vi "Box Function.vi"(6 "Index":i32, 9 "Freq Index":u8, 10 "Signal Type":enum16{"Sine", "Square", "Triangle"}(ring), 11 "CAN Frame [Write] In":cluster{"Identifier":u32, "Data Bytes":u8[]} {"Data Bytes" format="%x"; "Identifier" format="%x"}) -> (1 "State":T1, 2 "Freq":dbl, 3 "CAN Frame [Write]":T2 {"payload" format="%x"; "timestamp" format="%<%I:%M:%S%8u %p\n%x>T"; "identifier" format="%x"})   [LabVIEW 2015]
uses:
  <vilib>/Stratom, Inc/X-CAN for myRIO (API)/X-CAN Class/Type Definitions/CANFrame.ctl
  Control/State.ctl
  <vilib>/Stratom, Inc/X-CAN for myRIO (API)/X-CAN Class/X-CAN.lvclass
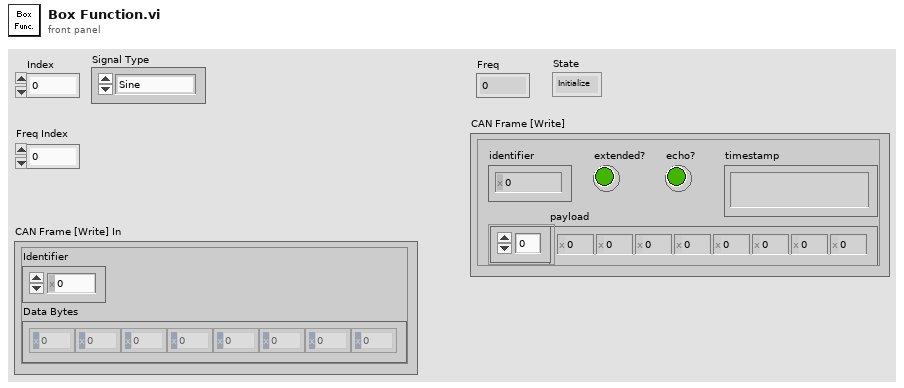
[diagram p1: front panel]
types:
  T1 = typedef "State.ctl" = enum16{"Initialize", "Idle", "Write", "Stop"}
  T2 = typedef "X-CAN.lvclass/CANFrame.ctl" = cluster{"identifier":u32, "extended?":bool, "echo?":bool, "payload":u8[], "timestamp":timestamp}
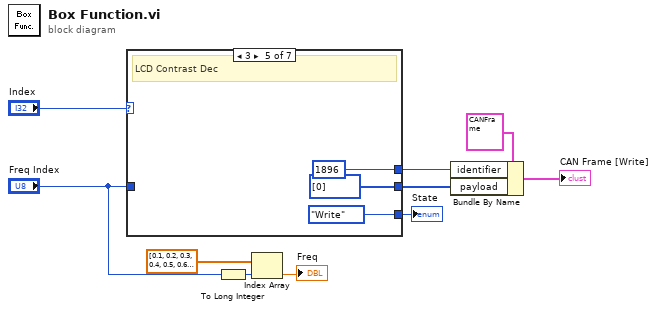
[diagram p0: block diagram]
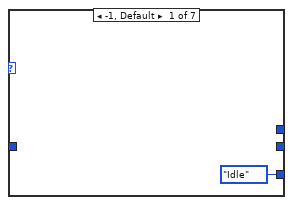
[diagram p2: hidden frame]
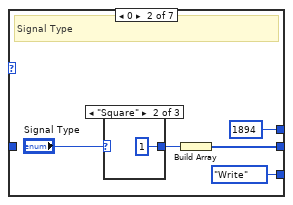
[diagram p3: hidden frame]
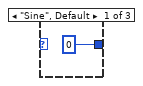
[diagram p4: hidden frame]
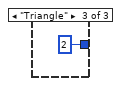
[diagram p5: hidden frame]
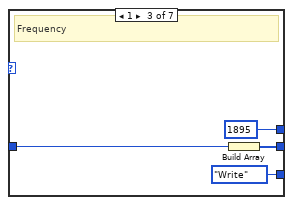
[diagram p6: hidden frame]
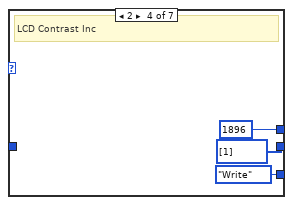
[diagram p7: hidden frame]
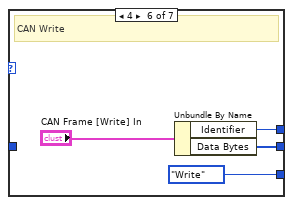
[diagram p8: hidden frame]
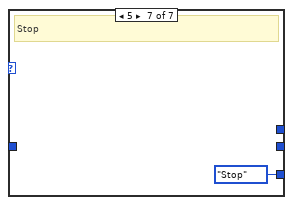
[diagram p9: hidden frame]
diagram:
  n1 = case shown="3" "Index" {
    tunnel: [_ u32 1894 u32 1895 u32 1896 u32 1896 w32 _] -> w7
    tunnel: [_ w13 w22 u8[] [1] ("Data Bytes") u8[] [0] ("Data Bytes") w31 _] -> w6
    tunnel: [State."Idle" State."Write" State."Write" State."Write" State."Write" State."Write" State."Stop"] -> w5
    tunnel: "Freq Index" -> [_ _ w20 _ _ _ _]
    frame -1, Default {
    }
    frame 0 {
      # "Signal Type"
      n2 = case shown="\"Square\"" "Signal Type" {
        tunnel: [u8 0 u8 1 u8 2] -> w14
        frame "Sine", Default {
        }
        frame "Square" {
        }
        frame "Triangle" {
        }
      }
      n3 = Build Array(w14) -> (w13:u8[])
    }
    frame 1 {
      # "Frequency"
      n4 = Build Array(w20) -> (w22:u8[])
    }
    frame 2 {
      # "LCD Contrast Inc"
    }
    frame 3 {
      # "LCD Contrast Dec"
    }
    frame 4 {
      # "CAN Write"
      n5 = Unbundle By Name("CAN Frame [Write] In") -> ("Identifier"=w32:u32, "Data Bytes"=w31:u8[])
    }
    frame 5 {
      # "Stop"
    }
  }
  "State" <- w5
  n6 = To Long Integer(number="Freq Index") -> (32bit integer=w3:i32)
  n7 = Index Array(array=dbl[] [0.1, 0.2, 0.3, 0.4, 0.5, 0.6, 0.7, 0.8, 0.9, 1.0, 2.0, 3.0, 4.0, 5.0, 6.0, 7.0, 8.0, 9.0, 10.0, 20.0, 30.0, 40.0, 50.0, 60.0, 70.0, 80.0, 90.0, 100.0, 110.0, 120.0, 130.0, 140.0, 150.0, 160.0, 170.0, 180.0, 190.0, 200.0, 210.0, 220.0, 230.0, 240.0, 250.0, 260.0, 270.0, 280.0, 290.0, 300.0, 310.0, 320.0, 330.0, 340.0, 350.0, 360.0, 370.0, 380.0, 390.0, 400.0, 410.0, 420.0, 430.0, 440.0, 450.0, 460.0, 470.0, 480.0, 490.0, 500.0, 510.0, 520.0, 530.0, 540.0, 550.0, 560.0, 570.0, 580.0, 590.0, 600.0, 610.0, 620.0, 630.0, 640.0, 650.0, 660.0, 670.0, 680.0, 690.0, 700.0, 710.0, 720.0, 730.0, 740.0, 750.0, 760.0, 770.0, 780.0, 790.0, 800.0, 810.0, 820.0, 830.0, 840.0, 850.0, 860.0, 870.0, 880.0, 890.0, 900.0, 910.0, 920.0, 930.0, 940.0, 950.0, 960.0, 970.0, 980.0, 990.0, 1000.0] ("appended array"), index=w3) -> (element=→"Freq":dbl)
  n8 = Bundle By Name(cluster=T2 {"identifier"=0, "extended?"=FALSE, "echo?"=FALSE, "payload"=[0, 0, 0, 0, 0, 0, 0, 0], "timestamp"=timestamp(0 s since 1904-01-01)} ("CAN Frame [Write]"), "identifier"=w7, "payload"=w6) -> (→"CAN Frame [Write]":T2)
